vi "error intake.vi"(10 "LabVIEW Object":refnum<class>, 11 "Template in":refnum<class "Template.lvclass">) -> ()   [LabVIEW 2020, in "Template.lvlib" / "Template.lvclass"]
doc: "This method decides either between seeking for an error handling nested actor or to forward the error to an upstream actor\nIf this is executed in the root actor, searches for an error handling module. If an error handling actor is not found, sends emergency stop to application.\nIf this method is executed in a nested actor, sends the error upstream by executing the process error interface override in the callers enqueuer as priority message"
uses:
  Template.lvclass
  C:/Program Files/National Instruments/LabVIEW 2020/vi.lib/ActorFramework/Actor/Actor.lvclass
  <vilib>/ActorFramework/Actor/Actor.lvclass/Actor.ctl
  Template Messages/fire error object Msg/fire error object Msg.lvclass/fire error object Msg.ctl
  <vilib>/ActorFramework/Message Enqueuer/Message Enqueuer.lvclass/Message Enqueuer.ctl
  Template.lvclass/Template.ctl
  <vilib>/ActorFramework/Message Enqueuer/Message Priority.ctl
  Template Messages/process error Msg/process error Msg.lvclass/process error Msg.ctl
  <vilib>/ActorFramework/Message Enqueuer/Equals Not A Refnum.vi
  <vilib>/ActorFramework/Actor/Read Caller Enqueuer.vi
  Template Messages/fire error object Msg/Send fire error object.vi
  <vilib>/ActorFramework/Message Enqueuer/Init from Existing Queue.vi
  <vilib>/ActorFramework/Message Enqueuer/Enqueue.vi
  Template Messages/fire error object Msg/fire error object Msg.lvclass
  C:/Program Files/National Instruments/LabVIEW 2020/vi.lib/ActorFramework/Message/Message.lvclass
  Template Messages/process error Msg/process error Msg.lvclass
  <vilib>/ActorFramework/Message Priority Queue/Priority Enqueue.vi
  <vilib>/ActorFramework/Message Enqueuer/Message Enqueuer.lvclass
  interfaces/Error Interface/Error/Error.lvclass
  <vilib>/ActorFramework/Actor/Actor.lvclass
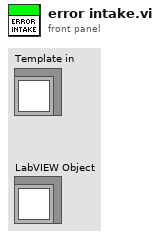
[diagram p1: front panel]
types:
  T1 = typedef "Actor Framework.lvlib/Message Enqueuer.lvclass/Message Priority.ctl" = enum16{"Low", "Normal", "High"}
  T2 = map{string, refnum<class "Message Enqueuer.lvclass">}
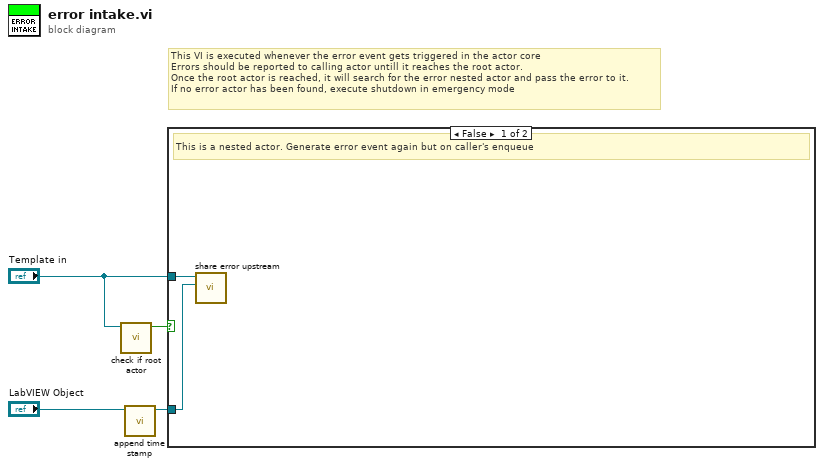
[diagram p0: block diagram]
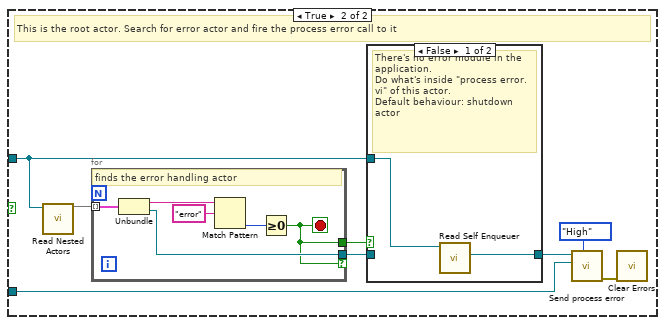
[diagram p2: hidden frame]
diagram:
  # "This VI is executed whenever the error event gets triggered in the actor core\nErrors should be reported to calling actor untill it reaches the root actor.\nOnce the root actor is reached, it will search for the error nested actor and pass the error to it.\nIf no error actor has been found, execute shutdown in emergency mode"
  n1 = call "check if root actor.vi"("Template in"="Template in") -> ("Is Root Actor?"=w4:bool)  [unwired: 10 in]
  n2 = call "append time stamp.vi"("Error in"="LabVIEW Object") -> ("Error out"=w1:refnum<class "Error.lvclass">)  [unwired: 10 in]
  n3 = case shown="False" w4 {
    tunnel: "Template in" -> [w6 w12]
    tunnel: w1 -> [w5 w7]
    frame False {
      # "This is a nested actor. Generate error event again but on caller's enqueue"
      n4 = call "share error upstream.vi"("Error Object"=w5, "Template in"=w6) -> ()  [unwired: 10 in]
    }
    frame True {
      # "This is the root actor. Search for error actor and fire the process error call to it"
      n5 = call "Read Nested Actors.vi"("Template in"=w12) -> ("Nested Actors"=w14:T2)  [unwired: 10 in]
      n6 = for {
        tunnel: w14 -> [w23] mode=indexing
        tunnel: [w19] -> w11 if=w18
        tunnel: [w18] -> w13
        stop <- w18 stop-if-true
        # "finds the error handling actor"
        n7 = Unbundle(w23) -> (w22:string, "Nested Enqueuer"=w19:refnum<class "Message Enqueuer.lvclass">)
        n8 = Match Pattern(string=w22, regular expression="error") -> (offset past match=w20:i32)  [unwired: 1 in, 3 out]
        n9 = Greater Or Equal To 0?(x=w20) -> (x >= 0?=w18:bool)
      }
      n10 = case shown="False" w13 {
        tunnel: w12 -> [w16 _]
        tunnel: w11 -> [_ w17]
        tunnel: [w15 w17] -> w9
        frame False {
          # "There's no error module in the application.\nDo what's inside \"process error.vi\" of this actor.\nDefault behaviour: shutdown actor"
          n11 = call <vilib>:"Read Self Enqueuer.vi"("Actor"=w16) -> ("Self Enqueuer"=w15:refnum<class "Message Enqueuer.lvclass">)  [unwired: 10 in]
        }
        frame True {
          # "Error module exists in the application.\nEnqueue \"process error.vi\" message in its enqueue"
        }
      }
      n12 = call "Send process error.vi"("Message Priority (Normal)"=Message_Priority."High", "Error Object"=w7, "Message Enqueuer"=w9) -> ("error out"=w8:errorcluster)  [unwired: 7 in, 1 out]
      n13 = call <vilib>:"Clear Errors.vi"("error in (no error)"=w8) -> ()  [unwired: 5 in, 2 out]
    }
  }
